vi "Easy2Acquire.vi"() -> (0 "Euler":dbl[][][](array[numeric]), 1 "MotionBuffer":dbl[][][](array[numeric]))   [LabVIEW 2017]
uses:
  MM-MotionSelect-CTRL.ctl
  <vilib>/picture/3D Picture Control/Object/Create Object (drawable).vi
  <vilib>/picture/3D Picture Control/Object/Add Object (reference).vi
  <vilib>/picture/3D Picture Control/NI_3D Picture Control.lvlib
panel:
  out "3DRef":refnum<vi>
  in  "stopcapture":bool
  in  "Set Analog Frequency":dbl=1500.0
  in  "Data":enum32{"Motion", "Analog", "Digital"}(tab)
  out "3D Picture":refnum<vi>(3d-picture)
  out "MotionChart":dbl[][](graph)
  in  "Motion.Select":T1
  out "AnalgoChart":dbl[][](graph)=[[-3.997772336006174, -9.006775449961426, -0.985625781118869, 32.99368263781076, 85.00003043934697, 76.99819933623077], [-2.008636832237248, 1.9934996329247954, 6.003357030451293, -20.0085451640189, 85.00003043934697, 75.99810778163375], [-0.9945677518844628, 7.998016599565745, 3.9873042963445156, 31.006439376622485, 86.99996940046543, 76.99819933623077], [-2.008636832237248, 6.989257749170066, 0.985625781118869, 162.001159552485, 86.99996940046543, 76.99819933623077], [-2.008636832237248, 6.00451696664095, 2.0160527341067773, 268.0056151561443, 88.00256347283715, 76.99819933623077], [-6.006409168243422, -3.002258483320475, 2.0160527341067773, 320.00061007216624, 88.00256347283715, 78.99838244542481], [-7.995544672012348, -4.011017333716155, 0.985625781118869, 404.00927725061837, 86.99996940046543, 76.99819933623077], [-9.009613752365134, -7.998016599565745, -0.985625781118869, 408.01098628342214, 88.99990836158389, 75.99810778163375], [-9.009613752365134, 6.00451696664095, 5.017731249332424, 260.00219709053675, 86.99996940046543, 75.99810778163375], [-9.009613752365134, 12.0090339332819, 3.9873042963445156, 65.98736527562151, 86.99996940046543, 77.99829089082779], [-18.994293928146405, 1.0087588503956797, 0.0, 31.986449752003004, 86.99996940046543, 76.99819933623077], [-17.00515842437748, -12.0090339332819, -3.0016785152256467, 62.01287875324497, 88.00256347283715, 76.99819933623077], [-17.00515842437748, -17.004792049527172, -6.003357030451293, 69.9890743084253, 86.99996940046543, 76.99819933623077], [-13.007386088371307, -9.991516232490541, -5.017731249332424, 73.01077296584856, 86.99996940046543, 75.99810778163375], [-10.004181504249596, 7.998016599565745, -0.985625781118869, 50.00775165483363, 86.99996940046543, 75.99810778163375], [2.008636832237248, 28.00506713241339, 0.0, 28.01196322962646, 85.00003043934697, 75.99810778163375], [2.008636832237248, 28.989807914942507, 5.017731249332424, -31.006439376622485, 86.0026245117187, 75.99810778163375], [7.995544672012348, 34.009584099054344, 3.9873042963445156, -167.99011184647705, 88.00256347283715, 75.99810778163375], [11.993317008018522, 37.01184258237482, 6.988982811570162, -235.99194289371408, 86.99996940046543, 74.99801622703673], [14.996521592140233, 26.99630828201771, 3.0016785152256467, -287.0069274343555, 86.99996940046543, 74.99801622703673], [21.002930760383656, 25.002808649092916, 3.9873042963445156, -310.00994874537037, 86.99996940046543, 75.99810778163375], [29.993043184280467, 26.99630828201771, 3.9873042963445156, -299.0120545327668, 88.00256347283715, 75.99810778163375], [27.009339928627078, 25.002808649092916, 3.0016785152256467, -310.00994874537037, 86.99996940046543, 74.99801622703673], [25.000703096389827, 22.00055016577244, 5.017731249332424, -242.98812807351388, 86.99996940046543, 73.99792467243971], [21.002930760383656, 9.006775449961426, 3.9873042963445156, -77.01248199865233, 86.99996940046543, 74.99801622703673], [13.007386088371307, -4.011017333716155, -0.985625781118869, 12.00512709841134, 88.00256347283715, 75.99810778163375], [6.006409168243422, -12.993774715811016, -3.0016785152256467, 66.99459816142927, 88.00256347283715, 76.99819933623077], [3.003204584121711, -20.991791315376762, -6.003357030451293, 107.99169886484759, 88.00256347283715, 75.99810778163375], [-3.997772336006174, -18.998291682451967, -6.003357030451293, 205.99273640289934, 86.99996940046543, 74.99801622703673], [-10.004181504249596, -18.998291682451967, -5.017731249332424, 299.0120545327668, 88.99990836158389, 74.99801622703673], [-27.009339928627078, -14.002533566206695, -0.985625781118869, 336.98745657876185, 86.99996940046543, 74.99801622703673], [-31.00711226463325, -3.002258483320475, 0.0, 313.0044248923664, 86.99996940046543, 73.99792467243971], [-32.00168001651771, 12.993774715811016, 6.003357030451293, 302.98654105514333, 86.99996940046543, 73.99792467243971], [-29.993043184280467, 36.00308373197914, 16.97964413836597, 261.989440351725, 86.99996940046543, 74.99801622703673], [-24.006135344505367, 42.992341481149204, 16.97964413836597, 106.00445560365931, 88.00256347283715, 73.99792467243971], [-27.009339928627078, 33.000825248658664, 11.021088279783717, -58.99118009582171, 88.00256347283715, 73.99792467243971], [-24.006135344505367, 15.011292416602375, 3.9873042963445156, -133.00918594747802, 88.00256347283715, 72.99783311784269], [-13.007386088371307, 4.011017333716155, 2.0160527341067773, -159.9866937808695, 86.99996940046543, 73.99792467243971], [3.997772336006174, -1.0087588503956797, 0.0, -175.9935299120846, 88.00256347283715, 74.99801622703673], [18.994293928146405, -6.989257749170066, -2.0160527341067773, -159.9866937808695, 88.00256347283715, 74.99801622703673], [21.002930760383656, -22.00055016577244, -6.988982811570162, -126.01300076767822, 88.00256347283715, 72.99783311784269], [35.00488460063942, -31.007325615733865, -12.006714060902587, -151.0032653398814, 90.99984732270235, 72.99783311784269], [40.99179244041452, -31.99206639826298, -9.99066132679581, -253.00601191073696, 88.99990836158389, 73.99792467243971], [39.0026569366456, -28.989807914942507, -6.988982811570162, -144.0070801600816, 88.00256347283715, 72.99783311784269], [31.00711226463325, -28.00506713241339, -6.988982811570162, -68.00183104723702, 88.00256347283715, 73.99792467243971], [20.00836300849919, -23.994049798697237, -5.017731249332424, -64.00012201443324, 88.00256347283715, 73.99792467243971], [17.999726176261944, -20.007050532847646, 0.985625781118869, -29.999206490814732, 88.00256347283715, 73.99792467243971], [25.000703096389827, 0.0, 6.988982811570162, -64.00012201443324, 88.00256347283715, 73.99792467243971], [25.000703096389827, 9.006775449961426, 9.00503554567694, -19.001312278211145, 88.00256347283715, 72.99783311784269], [15.991089344024696, 6.00451696664095, 8.019409764558072, -25.99749745801095, 88.00256347283715, 73.99792467243971]]
  in  "Analog.Select":T1
  out "DigitalChart":dbl[][](graph)
  in  "Digital.Select":T1
  in  "endprogram":bool
  in  "startcapture":bool
  in  "connect":bool
  out "hardwaresetup?":bool
  out "GetComponentCount":i32
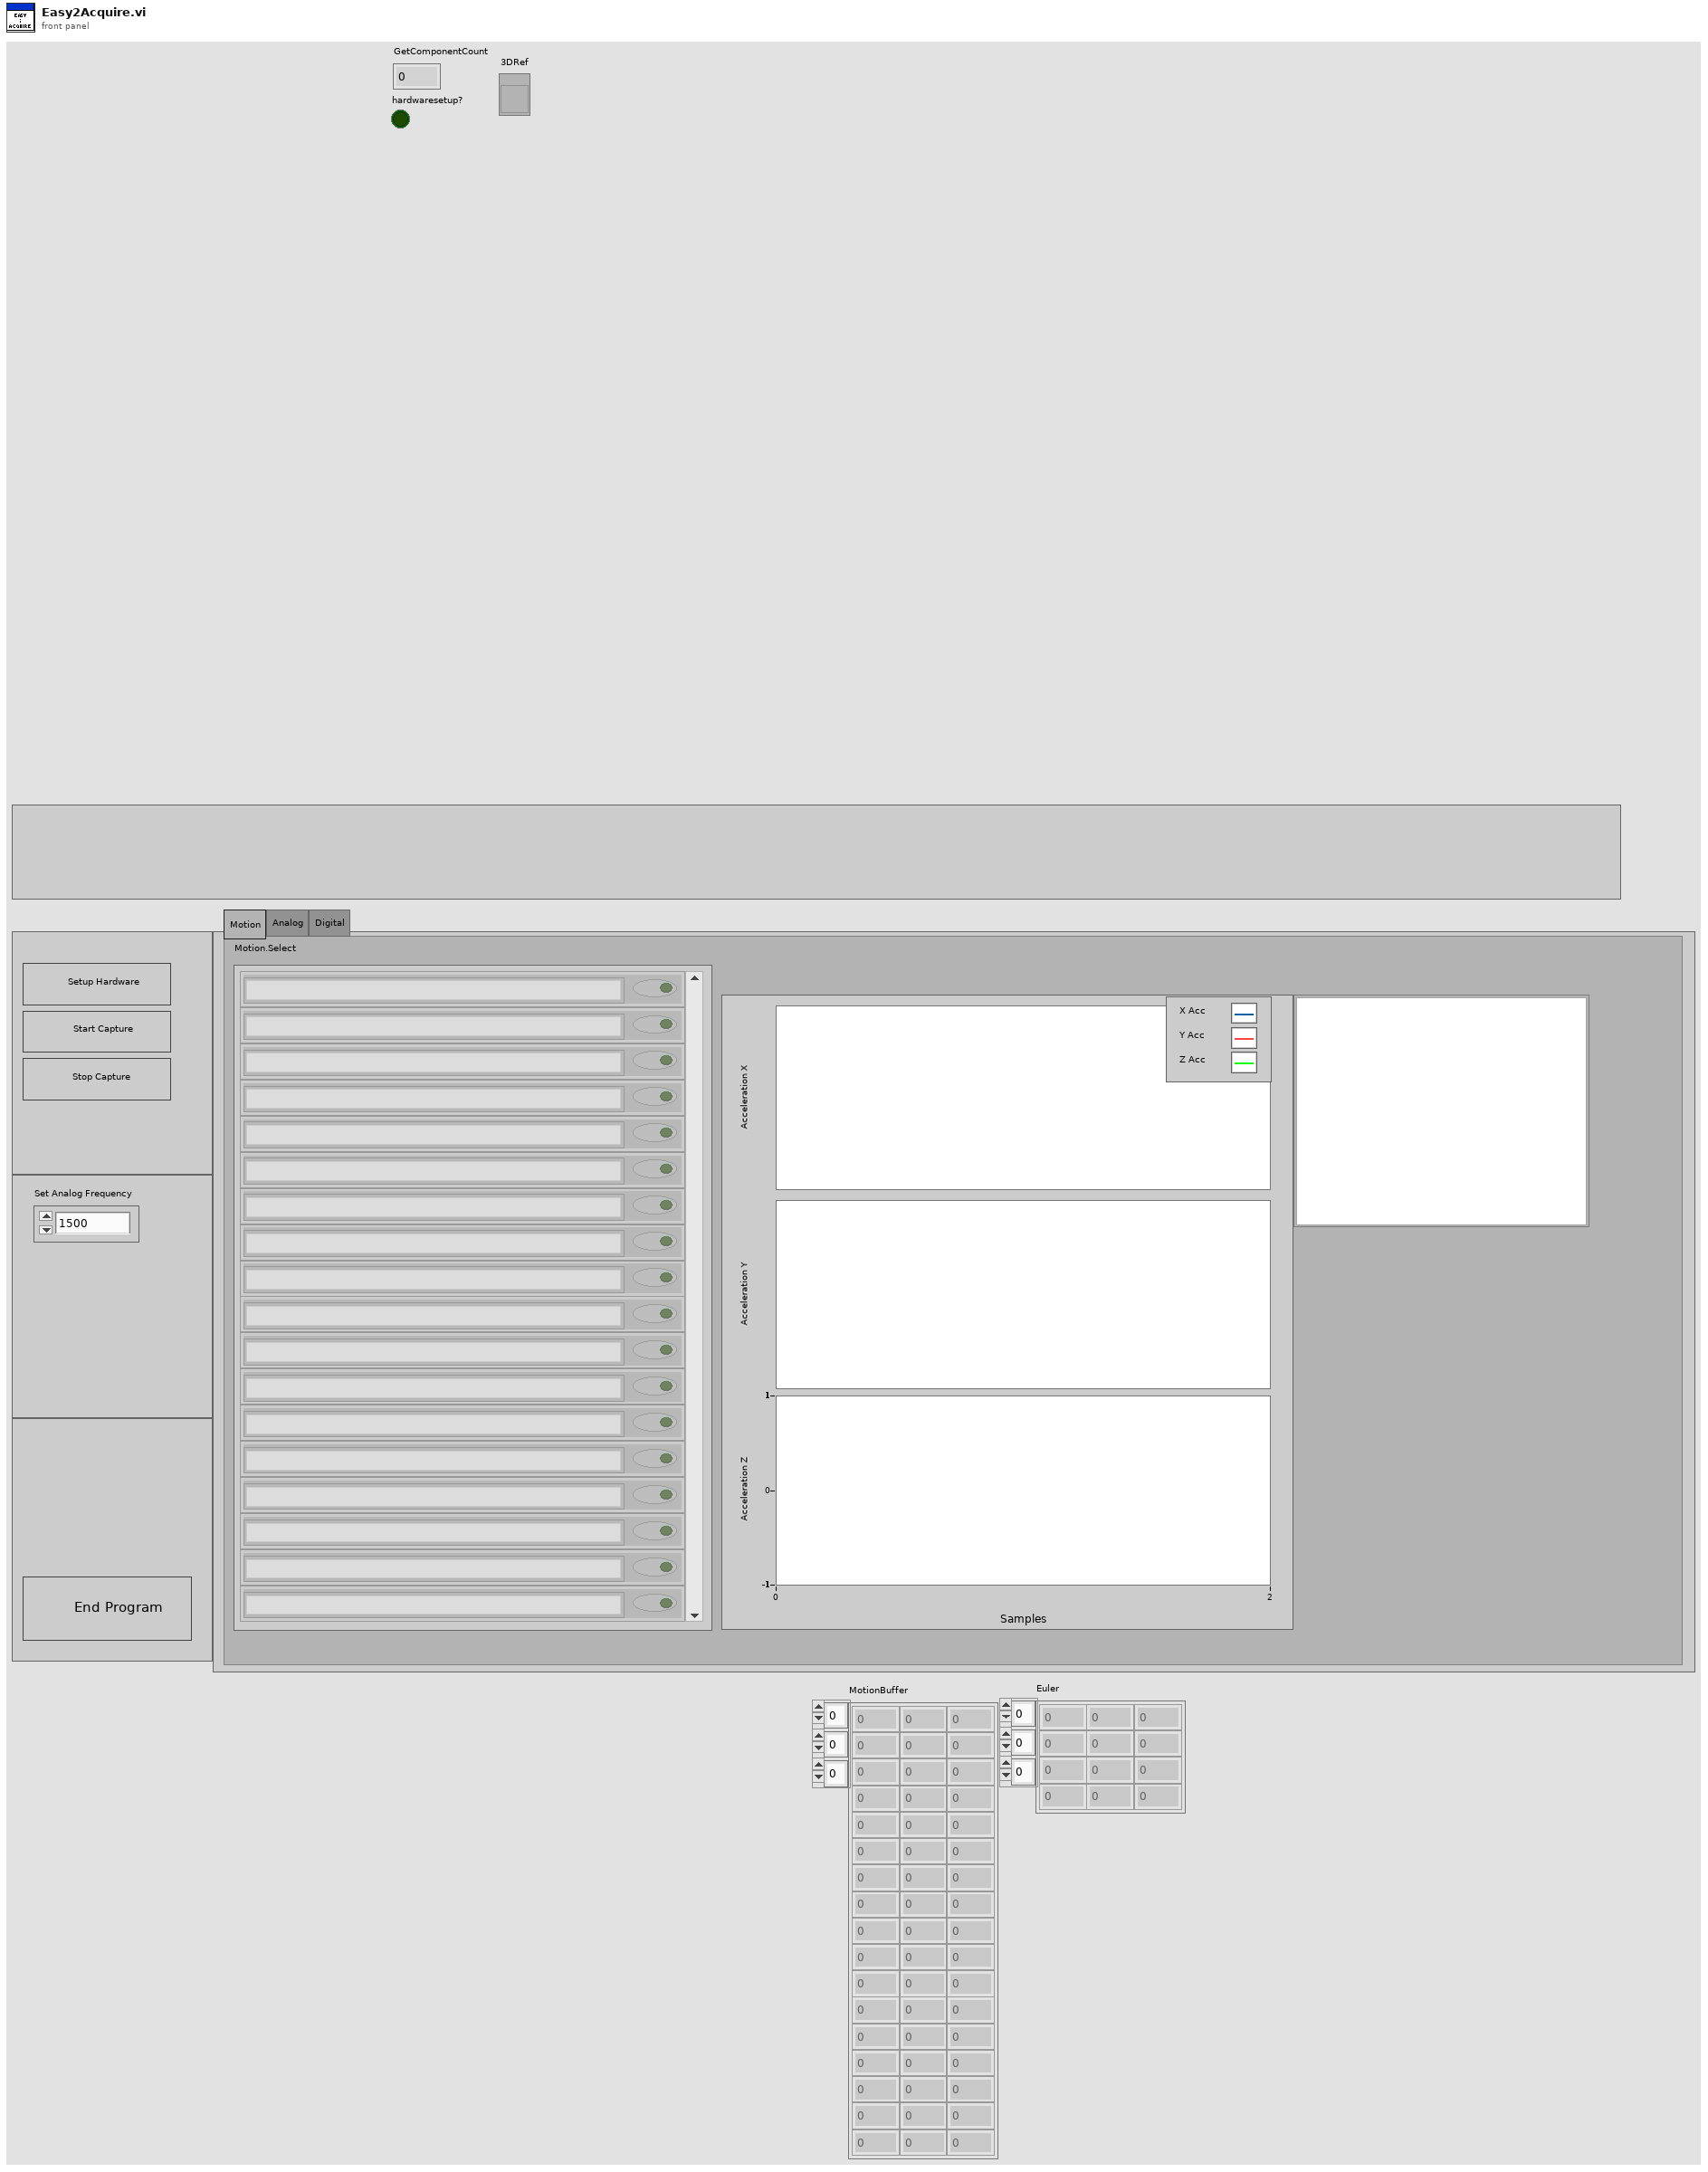
[diagram p1: front panel]
types:
  T1 = typedef "MM-MotionSelect-CTRL.ctl" = cluster{"Component":string, "Collect":bool}[]
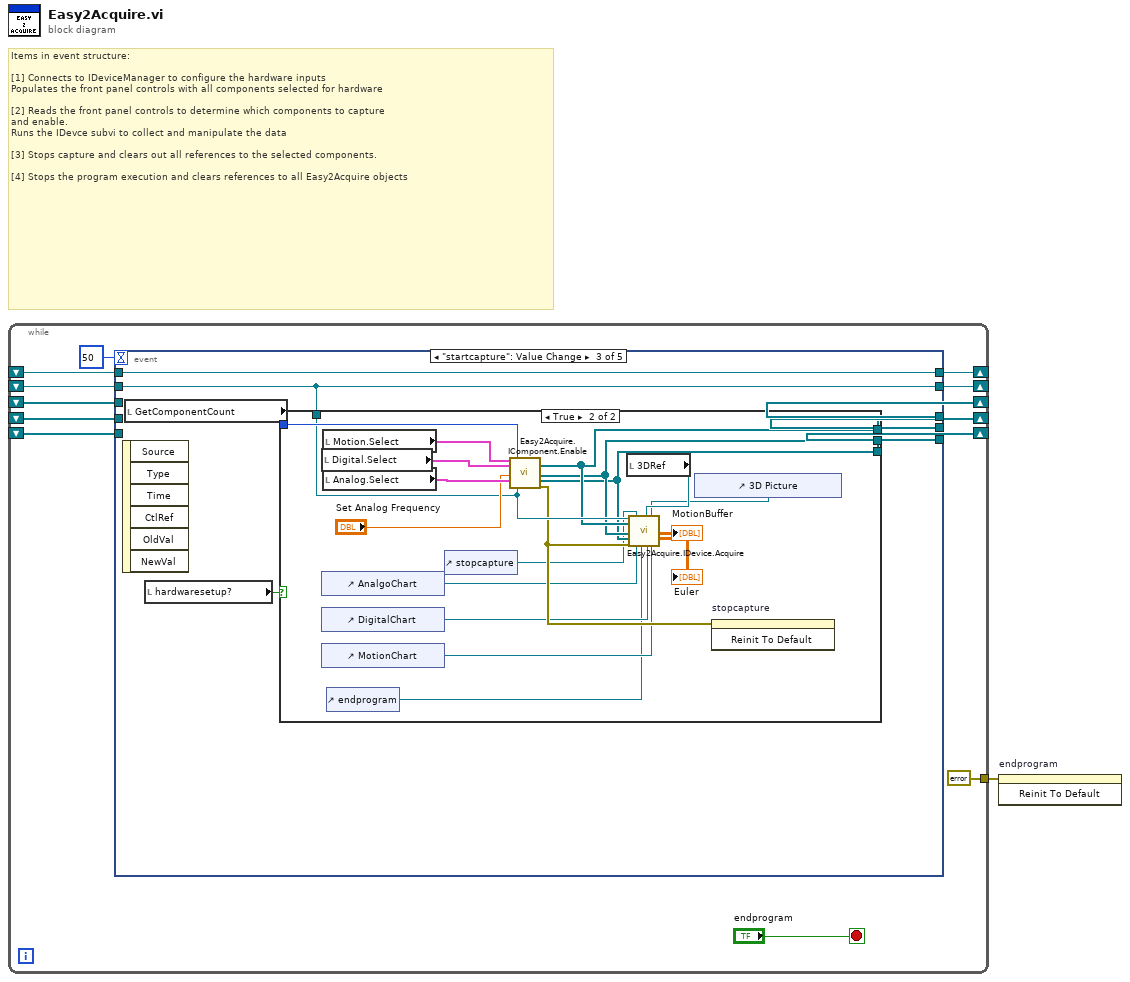
[diagram p0: block diagram]
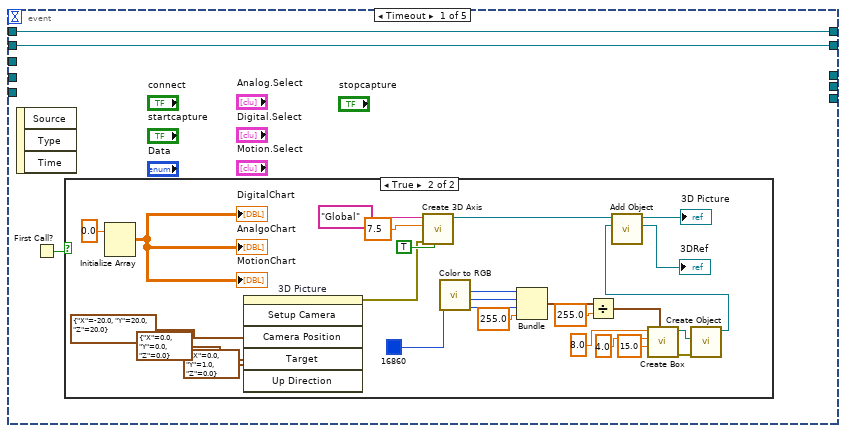
[diagram p2: hidden frame]
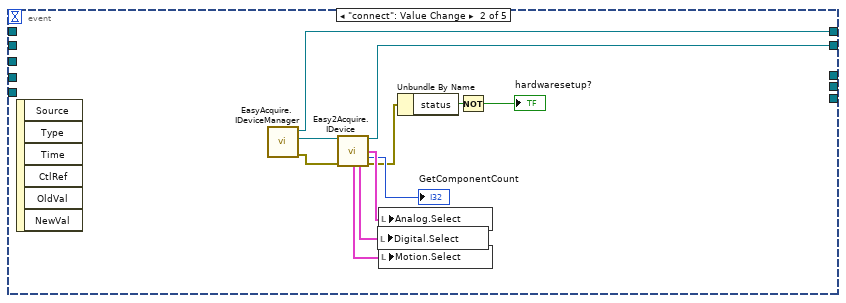
[diagram p4: hidden frame]
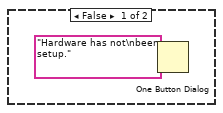
[diagram p5: hidden frame]
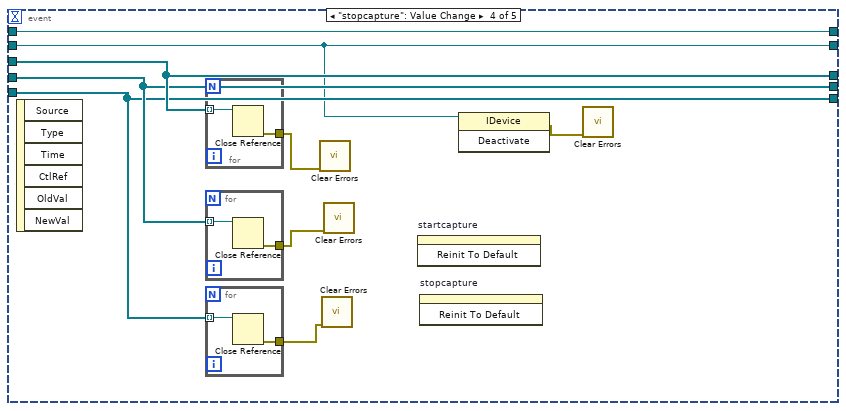
[diagram p6: hidden frame]
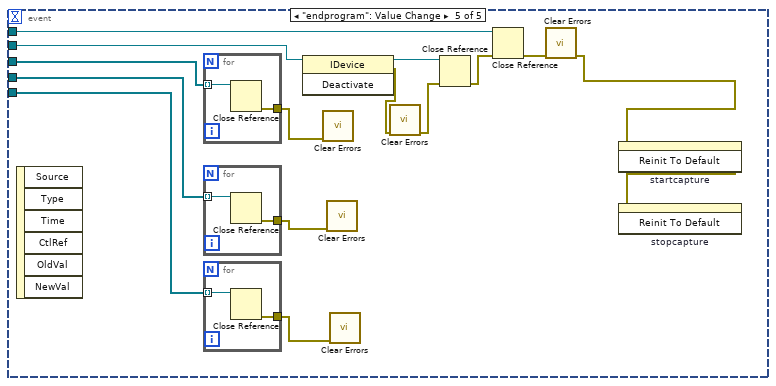
[diagram p7: hidden frame]
diagram:
  # "Items in event structure:\n\n[1] Connects to IDeviceManager to configure the hardware inputs \nPopulates the front panel controls with all components selected for hardware\n\n[2] Reads the front panel controls to determine which components to capture\nand enable.\nRuns the IDevce subvi to collect and manipulate the data\n\n[3] Stops capture and clears out all references to the selected components.\n\n[4] Stops the program execution and clears references to all Easy2Acquire objects"
  n1 = while {
    shift-right: [w12] -> _
    shift-left: _ -> [w11]
    shift-right: [w10] -> _
    shift-left: _ -> [w9]
    shift-right: [w8] -> _
    shift-left: _ -> [w5]
    shift-right: [w7] -> _
    shift-left: _ -> [w4]
    shift-right: [w6] -> _
    shift-left: _ -> [w3]
    tunnel: [errorcluster {"status"=FALSE, "code"=0, "source"=""} ("error constant")] -> w1
    stop <- "endprogram" stop-if-true
    n2 = event shown="[2] \"startcapture\": Value Change" {
      selector: _ -> [_ _ _ _ _]
      dyn-events: _ -> [_ _ _ _ _]
      timeout: 50 -> [_ _ _ _ _]
      tunnel: [w17 w50 w58 w86 _] -> w12
      tunnel: w11 -> [w17 _ w58 w86 w105]
      tunnel: [w16 w49 w61 w90 _] -> w10
      tunnel: w9 -> [w16 _ w61 w90 w111]
      tunnel: [_ _ w57 w89 _] -> w8
      tunnel: [_ _ w56 w88 _] -> w7
      tunnel: [_ _ w55 w87 _] -> w6
      tunnel: w5 -> [_ _ _ w89 w109]
      tunnel: w4 -> [_ _ _ w88 w108]
      tunnel: w3 -> [_ _ _ w87 w107]
      event Timeout {
        n3 = event-data() -> ()  [unwired: 1 in, 3 out]
        n4 = First Call?() -> (First Call?: T/F=w15:bool)
        n5 = case shown="True" w15 {
          frame False {
          }
          frame True {
            n6 = Initialize Array(0.0 ("element")) -> (→"DigitalChart" →"AnalgoChart" →"MotionChart":dbl[][])  [unwired: 2 in]
            n7 = invoke on="3D Picture" class="SceneGraphDisp (strict)" method="Setup Camera"("Camera Position"=cluster{"X":sgl, "Y":sgl, "Z":sgl} {"X"=-20.0, "Y"=20.0, "Z"=20.0}, "Target"=cluster{"X":sgl, "Y":sgl, "Z":sgl} {"X"=0.0, "Y"=0.0, "Z"=0.0}, "Up Direction"=cluster{"X":sgl, "Y":sgl, "Z":sgl} {"X"=0.0, "Y"=1.0, "Z"=0.0}) -> (error out=w23:errorcluster)  [unwired: 3 in, 5 out]
            n8 = call <vilib>:"Create 3D Axis.vi"("Axis label?"=TRUE, "error in (no error)"=w23, "Length"=sgl 7.5 ("Character Size"), "Name"="Global") -> ("New Object Refnum"=w27:refnum<vi>)  [unwired: 6 in, 1 out]
            n9 = call <vilib>:"Color to RGB.vi"("Color"=u32 16860 ("Color Box")) -> ("R"=w33:u8, "G"=w34:u8, "B"=w35:u8)  [unwired: 1 out]
            n10 = Bundle("R"=w33, "G"=w34, "B"=w35, 255.0) -> (w37:cluster{"R":u8, "G":u8, "B":u8, dbl})  [unwired: 1 in]
            n11 = Divide(x=w37, y=255.0) -> (x/y=w39:cluster{"R":dbl, "G":dbl, "B":dbl, dbl})
            n12 = call <vilib>:"Create Box.vi"("Color"=w39, "Length Z"=sgl 15.0, "Length Y"=sgl 4.0 ("Radius"), "Length X"=sgl 8.0 ("Height")) -> ("error out"=w30:errorcluster, "New Box Refnum"=w29:refnum<vi>)  [unwired: 6 in]
            n13 = call-poly <vilib>:"Create Object.vi"("error in (no error)"=w30, "Geometry"=w29) -> ("Scene:New Object"=w26:refnum<vi>)  [unwired: 8 in, 1 out]
            n14 = call-poly <vilib>:"Add Object.vi"("New Object In"=w26, "Scene Object In"=w27) -> ("New Object Out"=→"3DRef":refnum<vi>, "Scene Object Out"=→"3D Picture":refnum<vi>)  [unwired: 7 in, 1 out]
          }
        }
      }
      event "connect": Value Change {
        n15 = event-data() -> ()  [unwired: 1 in, 6 out]
        n16 = call "EasyAcquire.IDeviceManager.vi"() -> ("error out"=w47:errorcluster, "GetCurrentDevice"=w54:refnum<k7>, "Automation Refnum out"=w49:refnum<k7>)  [unwired: 8 in, 1 out]
        n17 = call "Easy2Acquire.IDevice.vi"("IDeviceIn"=w54, "error in"=w47) -> ("IDeviceOut"=w50:refnum<k7>, "Analog.Select"=w53:T1, "GetComponentCount"=→"GetComponentCount":i32, "Motion.Select"=w51:T1, "Digital.Select"=w52:T1, "error out"=w46:errorcluster)  [unwired: 8 in]
        n18 = local write "Digital.Select"(w52) -> ()
        n19 = local write "Analog.Select"(w53) -> ()
        n20 = local write "Motion.Select"(w51) -> ()
        n21 = Unbundle By Name(w46) -> ("status"=w45:bool)
        n22 = Not(x=w45) -> (.not. x?=→"hardwaresetup?":bool)
      }
      event "startcapture": Value Change {
        n23 = event-data() -> ()  [unwired: 1 in, 6 out]
        n24 = local read "GetComponentCount"() -> (w59:i32)
        n25 = local read "hardwaresetup?"() -> (w60:bool)
        n26 = case shown="True" w60 {
          tunnel: w59 -> [_ w78]
          tunnel: w58 -> [_ w76]
          tunnel: [_ w75] -> w57
          tunnel: [_ w74] -> w56
          tunnel: [_ w73] -> w55
          frame False {
            n27 = One Button Dialog(message="Hardware has not\nbeen setup.") -> ()  [unwired: 1 in, 1 out]
          }
          frame True {
            n28 = local read "Digital.Select"() -> (w80:T1)
            n29 = control-ref of="AnalgoChart"() -> (w66:refnum<vi>)
            n30 = control-ref of="DigitalChart"() -> (w68:refnum<vi>)
            n31 = control-ref of="MotionChart"() -> (w69:refnum<vi>)
            n32 = local read "Motion.Select"() -> (w79:T1)
            n33 = local read "Analog.Select"() -> (w81:T1)
            n34 = control-ref of="endprogram"() -> (w67:refnum<vi>)
            n35 = control-ref of="stopcapture"() -> (w65:refnum<vi>)
            n36 = call "Easy2Acquire.IComponent.Enable.vi"("Motion.Select"=w79, "Digital.Select"=w80, "AnalogFreq"="Set Analog Frequency", "Analog.Select"=w81, "ComponentCount"=w78, "IDeviceIn"=w76) -> ("AnalogInput"=w75:refnum<k7>[], "DigitalInput"=w74:refnum<k7>[], "MotionInput"=w73:refnum<k7>[], "error out"=w72:errorcluster)  [unwired: 10 in]
            n37 = local read "3DRef"() -> (w71:refnum<vi>)
            n38 = control-ref of="3D Picture"() -> (w70:refnum<vi>)
            n39 = call "Easy2Acquire.IDevice.Acquire.vi"("IDeviceIn"=w76, "IAnalogInput"=w75, "DigitalInput"=w74, "MotionInput"=w73, "error in (no error)"=w72, "stopcapture"=w65, "AnalgoChart"=w66, "endprogram"=w67, "3DRef"=w71, "DigitalChart"=w68, "3D Picture"=w70, "MotionChart"=w69) -> ("MotionBuffer"=→"MotionBuffer":dbl[][][], "Euler"=→"Euler":dbl[][][])  [unwired: 4 in, 2 out]
            n40 = invoke on="stopcapture" class="Bool (strict)" method="Reinit To Default"(error in=w72) -> ()  [unwired: 2 in, 3 out]
          }
        }
      }
      event "stopcapture": Value Change {
        n41 = event-data() -> ()  [unwired: 1 in, 6 out]
        n42 = for {
          tunnel: w89 -> [w96] mode=indexing
          tunnel: [w95] -> w85
          n43 = Close Reference(reference=w96) -> (error out=w95:errorcluster)  [unwired: 1 in]
        }
        n44 = for {
          tunnel: w88 -> [w94] mode=indexing
          tunnel: [w93] -> w84
          n45 = Close Reference(reference=w94) -> (error out=w93:errorcluster)  [unwired: 1 in]
        }
        n46 = for {
          tunnel: w87 -> [w92] mode=indexing
          tunnel: [w91] -> w83
          n47 = Close Reference(reference=w92) -> (error out=w91:errorcluster)  [unwired: 1 in]
        }
        n48 = call <vilib>:"Clear Errors.vi"("error in (no error)"=w85) -> ()  [unwired: 5 in, 2 out]
        n49 = call <vilib>:"Clear Errors.vi"("error in (no error)"=w83) -> ()  [unwired: 5 in, 2 out]
        n50 = call <vilib>:"Clear Errors.vi"("error in (no error)"=w84) -> ()  [unwired: 5 in, 2 out]
        n51 = invoke on="startcapture" class="Bool" method="Reinit To Default"() -> ()  [unwired: 3 in, 3 out]
        n52 = invoke on="stopcapture" class="Bool (strict)" method="Reinit To Default"() -> ()  [unwired: 3 in, 3 out]
        n53 = invoke class="IDevice" method="Deactivate"(reference=w86) -> (error out=w82:errorcluster)  [unwired: 2 in, 2 out]
        n54 = call <vilib>:"Clear Errors.vi"("error in (no error)"=w82) -> ()  [unwired: 5 in, 2 out]
      }
      event "endprogram": Value Change {
        n55 = event-data() -> ()  [unwired: 1 in, 6 out]
        n56 = for {
          tunnel: w109 -> [w117] mode=indexing
          tunnel: [w116] -> w101
          n57 = Close Reference(reference=w117) -> (error out=w116:errorcluster)  [unwired: 1 in]
        }
        n58 = for {
          tunnel: w108 -> [w115] mode=indexing
          tunnel: [w114] -> w99
          n59 = Close Reference(reference=w115) -> (error out=w114:errorcluster)  [unwired: 1 in]
        }
        n60 = for {
          tunnel: w107 -> [w113] mode=indexing
          tunnel: [w112] -> w100
          n61 = Close Reference(reference=w113) -> (error out=w112:errorcluster)  [unwired: 1 in]
        }
        n62 = invoke class="IDevice" method="Deactivate"(reference=w105) -> (reference out=w104:refnum<k7>, error out=w103:errorcluster)  [unwired: 2 in, 1 out]
        n63 = call <vilib>:"Clear Errors.vi"("error in (no error)"=w101) -> ()  [unwired: 5 in, 2 out]
        n64 = call <vilib>:"Clear Errors.vi"("error in (no error)"=w99) -> ()  [unwired: 5 in, 2 out]
        n65 = call <vilib>:"Clear Errors.vi"("error in (no error)"=w100) -> ()  [unwired: 5 in, 2 out]
        n66 = call <vilib>:"Clear Errors.vi"("error in (no error)"=w103) -> ("error out"=w102:errorcluster)  [unwired: 5 in, 1 out]
        n67 = Close Reference(reference=w104, error in (no error)=w102) -> (error out=w110:errorcluster)
        n68 = Close Reference(reference=w111, error in (no error)=w110) -> (error out=w106:errorcluster)
        n69 = call <vilib>:"Clear Errors.vi"("error in (no error)"=w106) -> ("error out"=w97:errorcluster)  [unwired: 5 in, 1 out]
        n70 = invoke on="startcapture" class="Bool" method="Reinit To Default"(error in=w97) -> (error out=w98:errorcluster)  [unwired: 2 in, 2 out]
        n71 = invoke on="stopcapture" class="Bool (strict)" method="Reinit To Default"(error in=w98) -> ()  [unwired: 2 in, 3 out]
      }
    }
  }
  n72 = invoke on="endprogram" class="Bool (strict)" method="Reinit To Default"(error in=w1) -> ()  [unwired: 2 in, 3 out]
